vi "test Modify Alias and Endpoint.vi"(8 "error in (no error)":errorcluster, 11 "TestCase in":refnum<class "Routing and Faulting Scripting Unit Tests.lvclass">) -> (0 "error out":errorcluster, 3 "TestCase out":refnum<class "Routing and Faulting Scripting Unit Tests.lvclass">)   [LabVIEW 2020, in "Routing and Faulting Scripting Unit Tests.lvclass"]
uses:
  Routing and Faulting Scripting Unit Tests.lvclass
  Shared/Alias Endpoint.ctl
  Routing and Faulting Scripting Unit Tests.lvclass/Routing and Faulting Scripting Unit Tests.ctl
  <vilib>/addons/_JKI Toolkits/VI Tester/TestCase.llb/TestCase.lvclass
  Routing and Faulting Scripting.lvlib
  Shared/Routing and Faulting Shared.lvlib
  C:/Program Files (x86)/National Instruments/LabVIEW 2020/vi.lib/addons/_JKI Toolkits/VI Tester/TestCase.llb/TestCase.lvclass
panel:
  in  "Save?":bool
  out "Output Filename":string
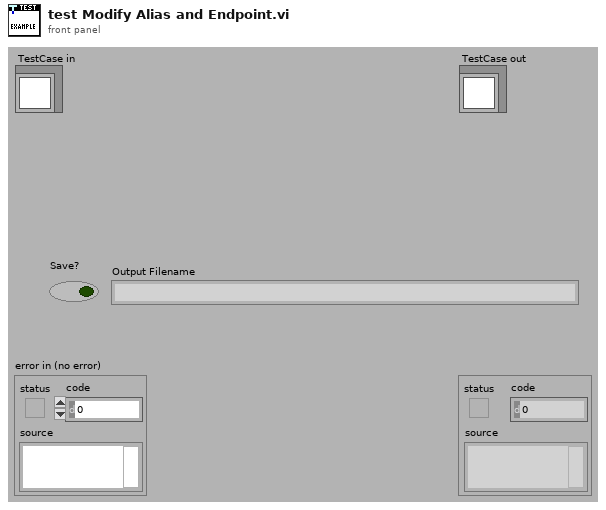
[diagram p1: front panel]
types:
  T1 = typedef "Routing and Faulting Shared.lvlib/Alias Endpoint.ctl" = cluster{"Module Path":string, "Endpoint":string}
  T2 = typedef "Custom Device API.lvlib/Custom Device Item Ref.ctl" = u64
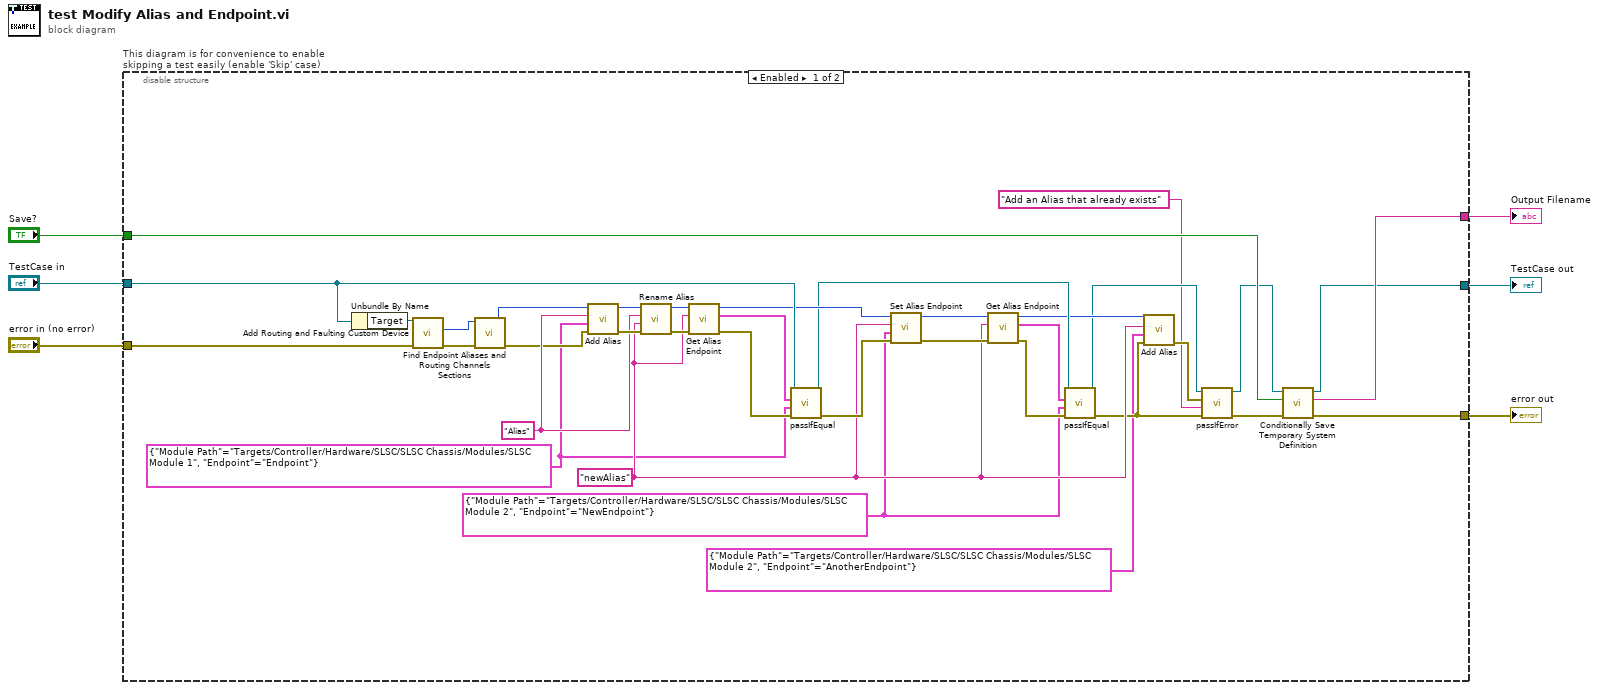
[diagram p0: block diagram]
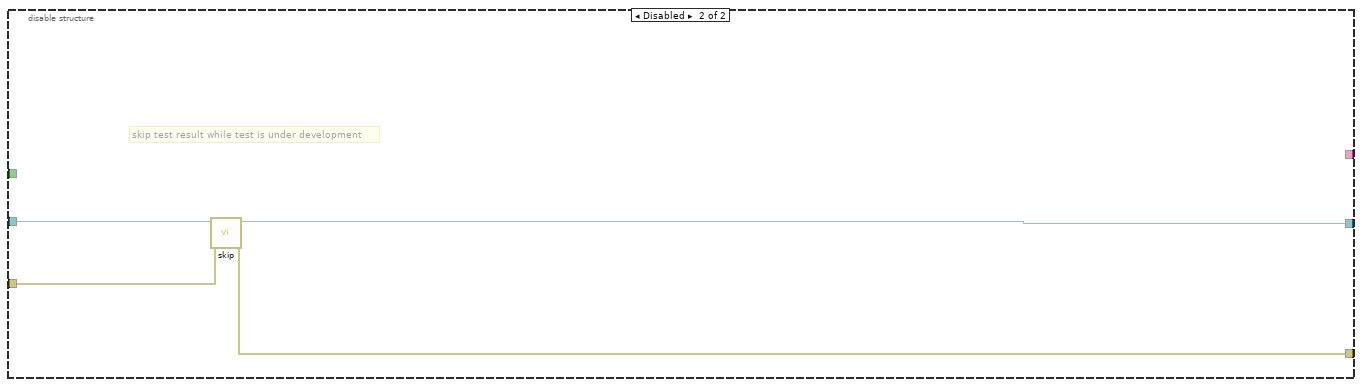
[diagram p2: hidden frame]
diagram:
  n1 = disable-structure "This diagram is for convenience to enable skipping a test easily (enable 'Skip' case)" shown="Enabled" {
    disable-tunnel: "TestCase in" -> [w37 w46]
    disable-tunnel: [w40 w44] -> w3
    disable-tunnel: [w41 w45] -> w5
    disable-tunnel: "error in (no error)" -> [w38 w43]
    disable-tunnel: [w42 _] -> w2
    disable-tunnel: "Save?" -> [w21 _]
    frame Enabled {
      w8 = T1 {"Module Path"="Targets/Controller/Hardware/SLSC/SLSC Chassis/Modules/SLSC Module 2", "Endpoint"="NewEndpoint"} ("Endpoint")
      w9 = T1 {"Module Path"="Targets/Controller/Hardware/SLSC/SLSC Chassis/Modules/SLSC Module 1", "Endpoint"="Endpoint"} ("Endpoint")
      w16 = "newAlias" ("Alias")
      w29 = "Alias" ("Alias")
      n2 = Unbundle By Name(w37) -> ("Target"=w39:refnum<k24>)
      n3 = call "Add Routing and Faulting Custom Device.vi"("error in"=w38, "target in"=w39) -> ("error out"=w36:errorcluster, "routing and faulting custom device"=w19:T2)  [unwired: 7 in, 1 out]
      n4 = call "Find Endpoint Aliases and Routing Channels Sections.vi"("error in"=w36, "routing and faulting custom device in"=w19) -> ("error out"=w20:errorcluster, "endpoint aliases"=w18:T2)  [unwired: 6 in, 2 out]
      n5 = call "Add Alias.vi"("error in"=w20, "endpoint"=w9, "alias"=w29, "endpoint aliases in"=w18) -> ("error out"=w31:errorcluster, "endpoint aliases out"=w33:T2)  [unwired: 6 in]
      n6 = call "Rename Alias.vi"("error in"=w31, "new alias name"=w16, "alias"=w29, "endpoint aliases in"=w33) -> ("error out"=w30:errorcluster, "endpoint aliases out"=w32:T2)  [unwired: 6 in]
      n7 = call "Get Alias Endpoint.vi"("error in"=w30, "alias"=w16, "endpoint aliases in"=w32) -> ("error out"=w34:errorcluster, "endpoint"=w35:T1, "endpoint aliases out"=w28:T2)  [unwired: 6 in]
      n8 = call-dynamic "passIfEqual.vi"("error in (no error)"=w34, "y"=w9, "x"=w35, "TestCase in"=w37) -> ("error out"=w27:errorcluster, "TestCase out"=w24:refnum<class "Routing and Faulting Scripting Unit Tests.lvclass">)  [unwired: 6 in]
      n9 = call "Set Alias Endpoint.vi"("error in"=w27, "new endpoint"=w8, "alias"=w16, "endpoint aliases in"=w28) -> ("error out"=w25:errorcluster, "endpoint aliases out"=w26:T2)  [unwired: 6 in]
      n10 = call "Get Alias Endpoint.vi"("error in"=w25, "alias"=w16, "endpoint aliases in"=w26) -> ("error out"=w22:errorcluster, "endpoint"=w23:T1, "endpoint aliases out"=w17:T2)  [unwired: 6 in]
      n11 = call-dynamic "passIfEqual.vi"("error in (no error)"=w22, "y"=w8, "x"=w23, "TestCase in"=w24) -> ("error out"=w14:errorcluster, "TestCase out"=w12:refnum<class "Routing and Faulting Scripting Unit Tests.lvclass">)  [unwired: 6 in]
      n12 = call "Add Alias.vi"("error in"=w14, "endpoint"=T1 {"Module Path"="Targets/Controller/Hardware/SLSC/SLSC Chassis/Modules/SLSC Module 2", "Endpoint"="AnotherEndpoint"} ("Endpoint"), "alias"=w16, "endpoint aliases in"=w17) -> ("error out"=w15:errorcluster)  [unwired: 6 in, 1 out]
      n13 = call-dynamic "passIfError.vi"("error in (no error)"=w14, "task (\"\")"="Add an Alias that already exists" ("task (\"\")"), "error"=w15, "TestCase in"=w12) -> ("error out"=w13:errorcluster, "TestCase out"=w11:refnum<class "Routing and Faulting Scripting Unit Tests.lvclass">)  [unwired: 6 in]
      n14 = call "Conditionally Save Temporary System Definition.vi"("error in (no error)"=w13, "Save?"=w21, "Test Case"=w11) -> ("error out"=w41:errorcluster, "filename"=w42:string, "Test Case"=w40:refnum<class "Routing and Faulting Scripting Unit Tests.lvclass">)  [unwired: 6 in]
    }
    frame Disabled {
      # "skip test result while test is under development"
      n15 = call <vilib>:"skip.vi"("error in (no error)"=w43, "TestCase in"=w46) -> ("error out"=w45:errorcluster, "TestCase out"=w44:refnum<class "Routing and Faulting Scripting Unit Tests.lvclass">)  [unwired: 8 in]
    }
  }
  "error out" <- w5
  "TestCase out" <- w3
  "Output Filename" <- w2
